vi "Mask Write Holding Register.vi"(4 "OR mask":u16, 6 "AND mask":u16, 8 "error in (no error)":errorcluster, 10 "address":u16, 11 "MB CR in":refnum<class "Modbus Master CR API.lvclass">) -> (0 "error out":errorcluster, 3 "MB CR out":refnum<class "Modbus Master CR API.lvclass">)   [LabVIEW 2021, in "Modbus Master CR API.lvclass"]
doc: "Writes values to one or more bits of a holding register."
uses:
  Modbus Master CR API.lvclass
  D:/my_projects/projects/Algorithms/Labview/21/Modbus_v121c/API/Modbus API.lvclass
  Modbus API.lvclass/Modbus API.ctl
  Network Protocol/MB/Modbus Master CR.lvclass/Modbus Master CR.ctl
  Read Network Protocol.vi
  Network Protocol/MB/Modbus Master CR.lvclass
  Data Model/Device Data Model.lvclass
  Modbus Master CR API.lvclass/Modbus Master CR API.ctl
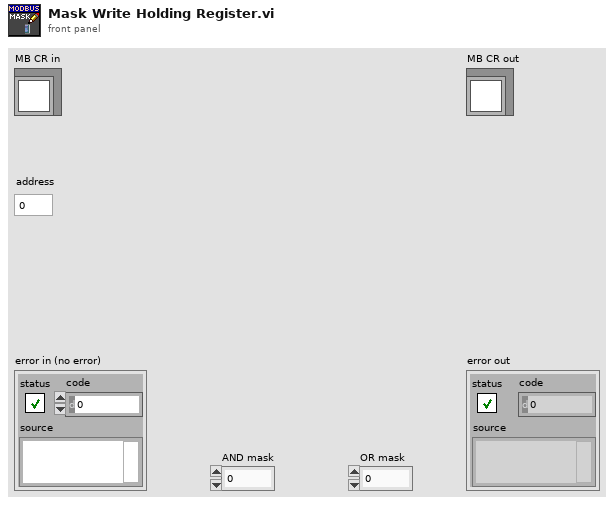
[diagram p1: front panel]
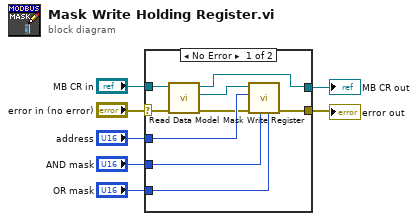
[diagram p0: block diagram]
diagram:
  n1 = case shown="No Error" "error in (no error)" {
    selector: "error in (no error)" -> [w12 w18]
    tunnel: [w16 w18] -> w6
    tunnel: "MB CR in" -> [w10 w17]
    tunnel: [w8 w17] -> w7
    tunnel: "address" -> [w15 _]
    tunnel: "AND mask" -> [w14 _]
    tunnel: "OR mask" -> [w13 _]
    frame No Error {
      n2 = call "Read Data Model.vi"("error in (no error)"=w12, "MB CR in"=w10) -> ("error out"=w11:errorcluster, "device data model"=w9:refnum<class "Device Data Model.lvclass">, "MB CR out"=w8:refnum<class "Modbus Master CR API.lvclass">)  [unwired: 7 in]
      n3 = call-dynamic "Mask Write Register.vi"("OR Mask"=w13, "AND Mask"=w14, "error in"=w11, "address"=w15, "device data model in"=w9) -> ("error out"=w16:errorcluster)  [unwired: 5 in, 1 out]
    }
    frame Error {
    }
  }
  "error out" <- w6
  "MB CR out" <- w7
